vi "Test CNV Log File.vi"() -> ()   [LabVIEW 2019]
uses:
  <vilib>/Utility/file.llb/Read Delimited Spreadsheet (DBL).vi
  <userlib>/_MGI/1D Array/MGI Calculate Array Differences/MGI Calculate Array Differences (DBL[]).vi
panel:
  out "Array":i32[](array[numeric])
  out "Waveform Chart":dbl[](graph)
  out "all rows":dbl[][](array[numeric])
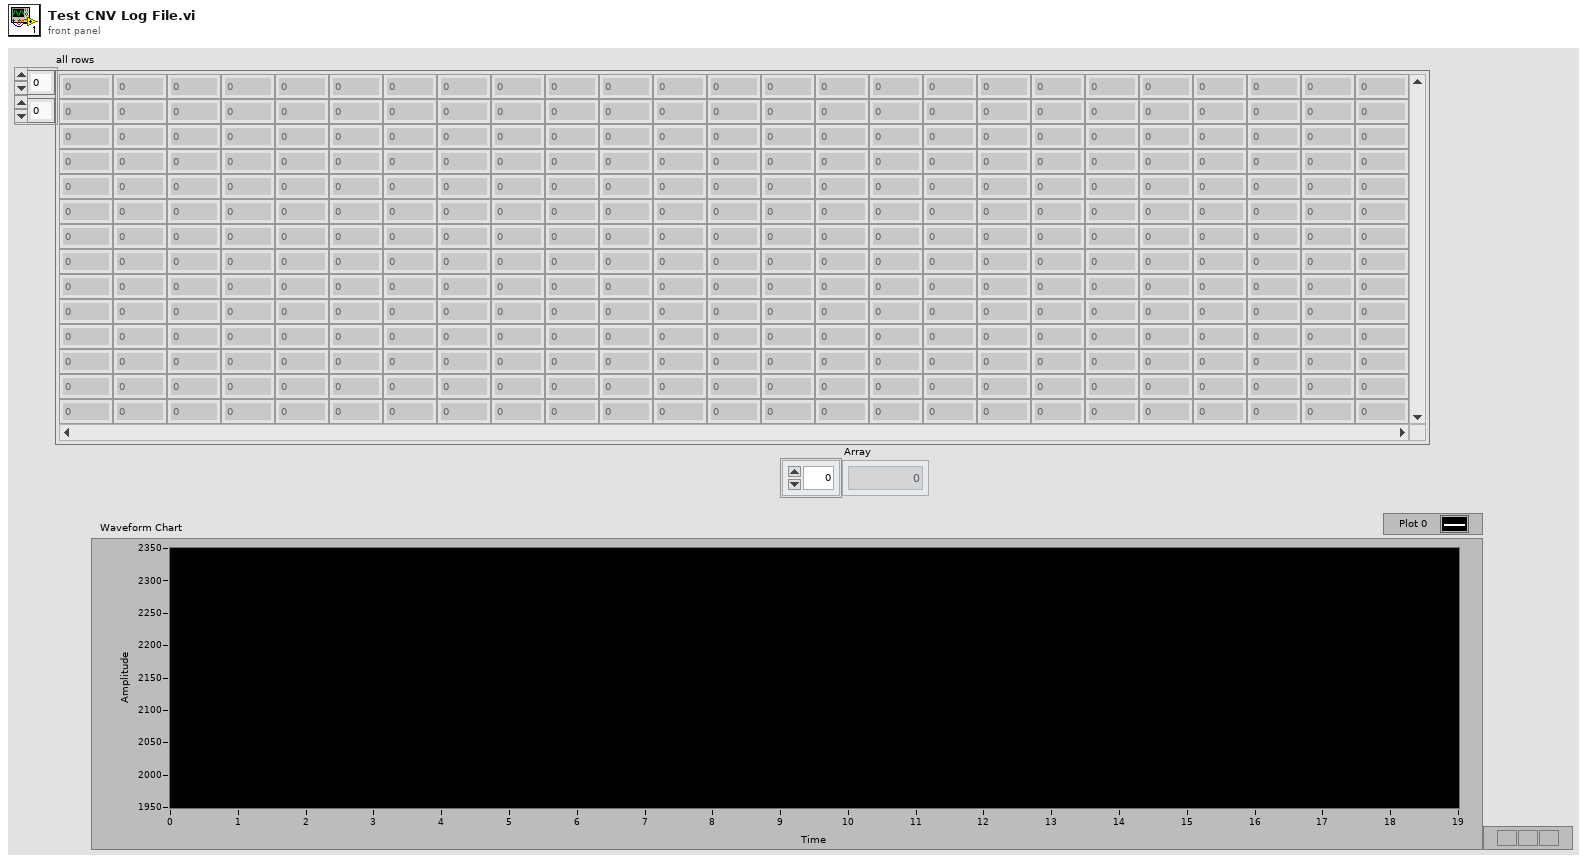
[diagram p1: front panel]
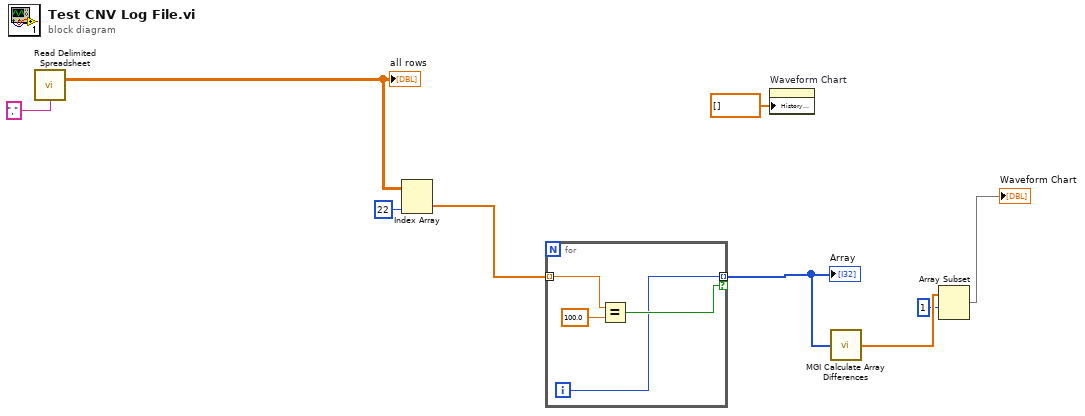
[diagram p0: block diagram]
diagram:
  n1 = call-poly <vilib>:"Read Delimited Spreadsheet.vi"("delimiter (\\t)"="," ("delimiter (\\t)")) -> ("all rows"=w8:dbl[][])  [unwired: 9 in, 5 out]
  "all rows" <- w8
  n2 = Index Array(array=w8, index (col)=22 ("disabled index (col)")) -> (element=w6:dbl[])  [unwired: 1 in]
  n3 = for {
    tunnel: w6 -> [w12] mode=indexing
    tunnel: [w10] -> w5 mode=indexing if=w11
    i -> [w10]
    n4 = Equal?(x=w12, y=100.0) -> (x = y?=w11:bool)
  }
  "Array" <- w5
  n5 = property on="Waveform Chart" class="WFChart (strict)"("History Data"=dbl[] []) -> ()  [unwired: 2 in, 2 out]
  n6 = call-poly <userlib>:"MGI Calculate Array Differences.vi"("x(i)"=w5) -> ("y(i)=x(i)-x(i-1)"=w4:dbl[])  [unwired: 1 in]
  n7 = Array Subset(array=w4, index=1) -> (→"Waveform Chart":dbl[])  [unwired: 1 in]
